vi "Close.vi"(11 "FpgaRef5782 In":refnum<class "FpgaRef5782.lvclass">) -> ()   [LabVIEW 2013, in "FpgaRef5782.lvclass"]
uses:
  FpgaRef5782.lvclass
  FpgaRefBase/FpgaRefBase.lvclass
  FpgaRef5782.lvclass/FpgaRef5782.ctl
  <vilib>/FPGAPlugInAG/Dynamic/niLvFpga_Close_Dynamic.vi
  <vilib>/rvi/interface/nirviCloseFPGA/nirviCloseFPGA.xnode
  5782 FPGA ref.ctl
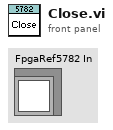
[diagram p1: front panel]
types:
  T1 = typedef "5782 FPGA ref.ctl" = refnum<k20>
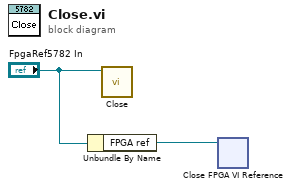
[diagram p0: block diagram]
diagram:
  n1 = Unbundle By Name("FpgaRef5782 In") -> ("FPGA ref"=w1:T1)
  n2 = call-parent "Close.vi"("FpgaRefBase In"="FpgaRef5782 In") -> ()  [unwired: 11 in]
  n3 = xnode "Close FPGA VI Reference"("FPGA VI Reference In"=w1) -> ()  [unwired: 1 in, 1 out]
